vi "Dequeue.vi"(8 "error in (no error)":errorcluster, 10 "create if not found? (f)":bool, 11 "ModuleAdmin":refnum<class "ModuleAdmin.lvclass">) -> (0 "error out":errorcluster, 1 "Message Data":variant, 2 "Message":string, 3 "ModuleAdmin Out":refnum<class "ModuleAdmin.lvclass">)   [LabVIEW 2014, in "SpecAnModule.lvlib"]
doc: "Dequeues a message and message data from a queue based on the queue name."
uses:
  SpecAnModule.lvlib
  <userlib>/NIST/ModuleAdminLib/ModuleAdmin/ModuleAdmin.lvclass
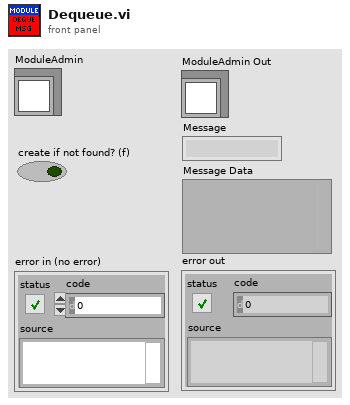
[diagram p1: front panel]
types:
  T1 = typedef "MyPluggableModule.lvlib/clMessage.ctl" = cluster{"Message":string, "Message Data":variant}
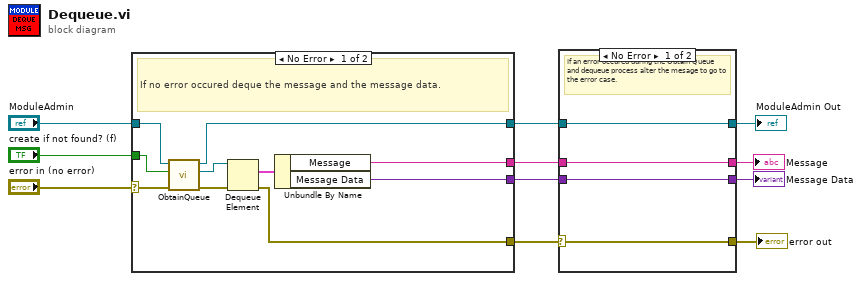
[diagram p0: block diagram]
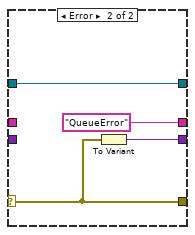
[diagram p2: hidden frame]
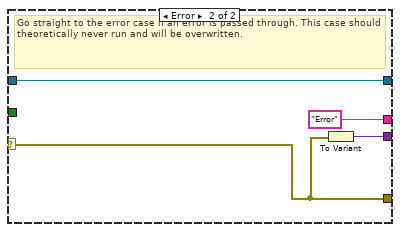
[diagram p3: hidden frame]
diagram:
  n1 = case shown="No Error" "error in (no error)" {
    selector: "error in (no error)" -> [w18 w23]
    tunnel: [w16 w25] -> w2
    tunnel: "ModuleAdmin" -> [w17 w25]
    tunnel: [w20 w23] -> w9
    tunnel: [w19 "Error" ("Message")] -> w6
    tunnel: "create if not found? (f)" -> [w13 _]
    tunnel: [w12 w22] -> w4
    frame No Error {
      # "If no error occured deque the message and the message data."
      n2 = call "ObtainQueue.vi"("error in (no error)"=w18, "create if not found? (f)"=w13, "ModuleAdmin"=w17) -> ("error out"=w15:errorcluster, "queue out"=w14:refnum<queue>, "ModuleAdmin Out"=w16:refnum<class "ModuleAdmin.lvclass">)  [unwired: 6 in]
      n3 = Dequeue Element(queue=w14, error in (no error)=w15) -> (element=w21:T1, error out=w20:errorcluster)  [unwired: 1 in, 2 out]
      n4 = Unbundle By Name(w21) -> ("Message"=w19:string, "Message Data"=w12:variant)
    }
    frame Error {
      # "Go straight to the error case if an error is passed through. This case should theoretically never run and will be overwritten."
      n5 = To Variant(anything=w23) -> (Variant=w22:variant)
    }
  }
  n6 = case shown="No Error" w9 {
    selector: w9 -> [w29 w32]
    tunnel: [w29 w32] -> w8
    tunnel: [w28 "QueueError" ("y")] -> w7
    tunnel: w6 -> [w28 _]
    tunnel: w4 -> [w27 _]
    tunnel: [w27 w31] -> w3
    tunnel: w2 -> [w26 w30]
    tunnel: [w26 w30] -> w1
    frame No Error {
      # "If an error occured during the Obtain Queue\nand dequeue process alter the mesage to go to\nthe error case."
    }
    frame Error {
      n7 = To Variant(anything=w32) -> (Variant=w31:variant)
    }
  }
  "error out" <- w8
  "ModuleAdmin Out" <- w1
  "Message" <- w7
  "Message Data" <- w3
